vi "Coord window-Normalise FOV for display.vi"(11 "Effective FOV (um)":sgl) -> (1 "Normalised Effective FOV/2":T1, 3 "Normalised Effective FOV":T2)   [LabVIEW 2013]
uses:
  Globals/Coord window-Globals.vi
  <vilib>/gmath/NI_Gmath.lvlib
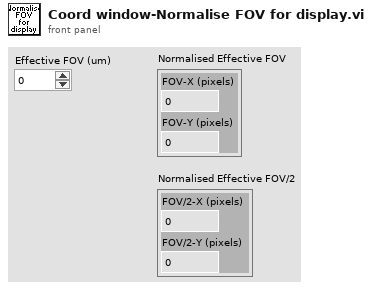
[diagram p1: front panel]
types:
  T1 = cluster{"FOV/2-X (pixels)":i16, "FOV/2-Y (pixels)":i16}
  T2 = cluster{"FOV-X (pixels)":i16, "FOV-Y (pixels)":i16}
  T3 = typedef "Coordinate list window refs.ctl" = cluster{"Window Name (i.e. Key)":string, "menu reference":refnum<k9>, "VI's reference":refnum<vi>, "Pane 1":refnum<vi>, "Pane 2":refnum<vi>, "Coord Listbox":refnum<vi>, "File name":refnum<vi>, "Picture Map":refnum<vi>, "Stage XYZ Position ind.":refnum<vi>}
  T4 = typedef "LVBoundsTypeDef.ctl" = cluster{"Width":u32, "Height":u32}
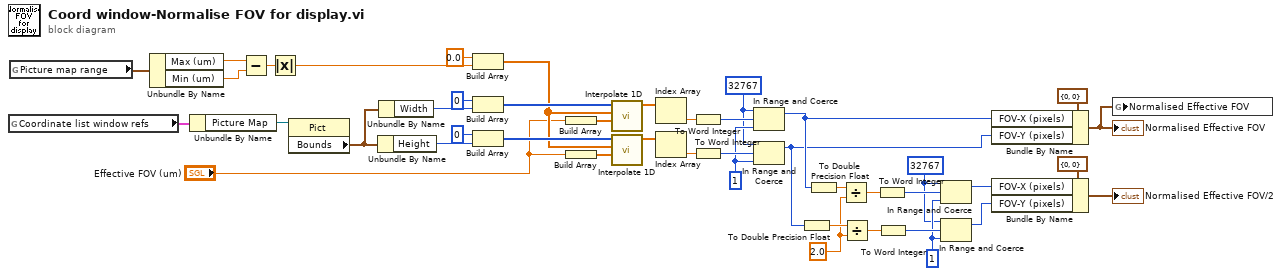
[diagram p0: block diagram]
diagram:
  w7 = i16 32767 ("lower limit")
  w9 = i16 1 ("lower limit")
  w8 = i16 32767 ("lower limit")
  w10 = i16 1 ("lower limit")
  w6 = 2.0 ("y")
  n1 = global read "Coord window-Globals.vi" "Coordinate list window refs"() -> (w32:T3)
  n2 = global read "Coord window-Globals.vi" "Picture map range"() -> (w38:cluster{"Min (um)":dbl, "Max (um)":dbl})
  n3 = Unbundle By Name(w38) -> ("Max (um)"=w15:dbl, "Min (um)"=w14:dbl)
  n4 = Unbundle By Name(w32) -> ("Picture Map"=w31:refnum<vi>)
  n5 = Subtract(x=w15, y=w14) -> (x-y=w13:dbl)
  n6 = Absolute Value(x=w13) -> (abs(x)=w12:dbl)
  n7 = property on="Property Node" class="Pict"(reference=w31) -> ("Bounds"=w30:T4)  [unwired: 1 in, 2 out]
  n8 = Unbundle By Name(w30) -> ("Height"=w42:u32)
  n9 = Unbundle By Name(w30) -> ("Width"=w39:u32)
  n10 = Build Array(0.0 ("element"), w12) -> (w37:dbl[])
  n11 = Build Array(u32 0 ("element"), w39) -> (w43:u32[])
  n12 = Build Array(u32 0 ("element"), w42) -> (w44:u32[])
  n13 = Build Array("Effective FOV (um)") -> (w36:sgl[])
  n14 = Build Array("Effective FOV (um)") -> (w33:sgl[])
  n15 = call <vilib>:"Interpolate 1D.vi"("xi"=w36, "X"=w37, "Y"=w43) -> ("yi"=w35:dbl[])  [unwired: 6 in, 2 out]
  n16 = call <vilib>:"Interpolate 1D.vi"("xi"=w33, "X"=w37, "Y"=w44) -> ("yi"=w34:dbl[])  [unwired: 6 in, 2 out]
  n17 = Index Array(array=w35) -> (element=w28:dbl)  [unwired: 1 in]
  n18 = Index Array(array=w34) -> (element=w27:dbl)  [unwired: 1 in]
  n19 = To Word Integer(number=w28) -> (16bit integer=w23:i16)
  n20 = To Word Integer(number=w27) -> (16bit integer=w16:i16)
  n21 = In Range and Coerce(upper limit=w8, x=w23, lower limit=w10) -> (coerced(x)=w5:i16)  [unwired: 1 out]
  n22 = In Range and Coerce(upper limit=w8, x=w16, lower limit=w10) -> (coerced(x)=w4:i16)  [unwired: 1 out]
  n23 = To Double Precision Float(number=w4) -> (double precision float=w21:dbl)
  n24 = To Double Precision Float(number=w5) -> (double precision float=w26:dbl)
  n25 = Divide(x=w26, y=w6) -> (x/y=w25:dbl)
  n26 = Divide(x=w21, y=w6) -> (x/y=w22:dbl)
  n27 = To Word Integer(number=w25) -> (16bit integer=w18:i16)
  n28 = To Word Integer(number=w22) -> (16bit integer=w17:i16)
  n29 = In Range and Coerce(upper limit=w7, x=w18, lower limit=w9) -> (coerced(x)=w3:i16)  [unwired: 1 out]
  n30 = In Range and Coerce(upper limit=w7, x=w17, lower limit=w9) -> (coerced(x)=w2:i16)  [unwired: 1 out]
  n31 = Bundle By Name(cluster=T2 {"FOV-X (pixels)"=0, "FOV-Y (pixels)"=0} ("Normalised Effective FOV"), "FOV-X (pixels)"=w5, "FOV-Y (pixels)"=w4) -> (w1:T2)
  "Normalised Effective FOV" <- w1
  n32 = Bundle By Name(cluster=T2 {"FOV-X (pixels)"=0, "FOV-Y (pixels)"=0} ("Normalised Effective FOV"), "FOV-X (pixels)"=w3, "FOV-Y (pixels)"=w2) -> (→"Normalised Effective FOV/2":T2)
  n33 = global write "Coord window-Globals.vi" "Normalised Effective FOV"(w1) -> ()
